vi "SetSamplingClockFrequency.vi"(1 "Sampling Clock Option":u16(ring) items=["Frequency Value", "Default", "Minimum", "Maximum"], 3 "error in (no error)":errorcluster, 4 "Sampling Clock (Hz)":dbl format="%#_16g", 5 "VISA resource name":refnum<visa-resource-name>) -> (0 "error out":errorcluster, 2 "VISA resource name out":refnum<visa-resource-name>)   [LabVIEW 2020, in "Active Technologies AWG3000.lvlib"]
uses:
  Active Technologies AWG3000.lvlib
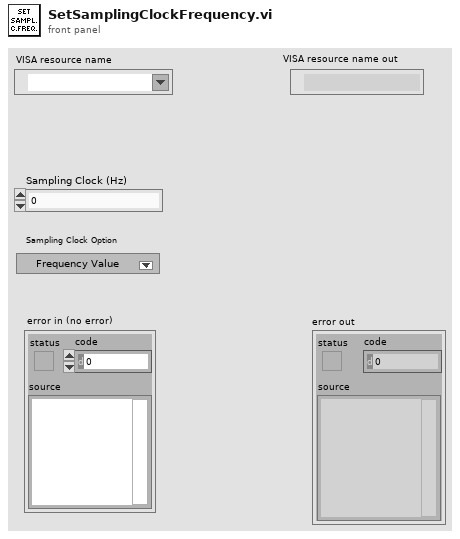
[diagram p1: front panel]
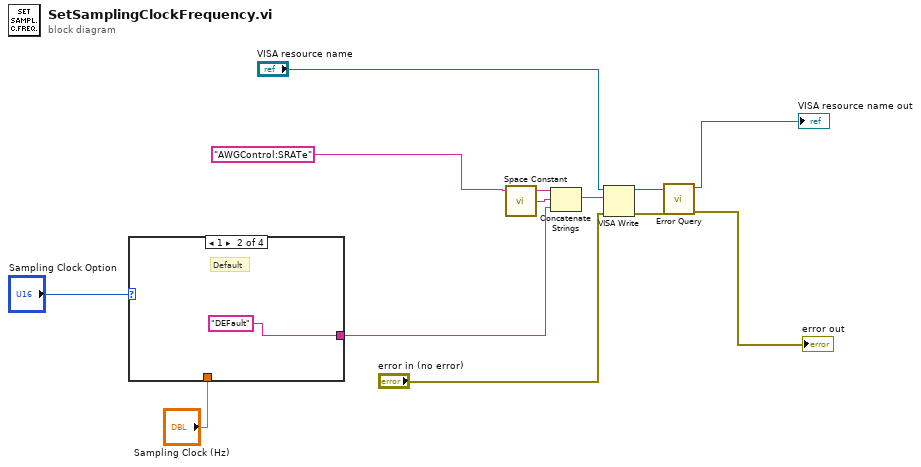
[diagram p0: block diagram]
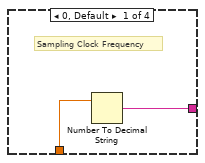
[diagram p2: hidden frame]
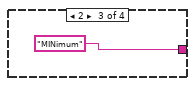
[diagram p3: hidden frame]
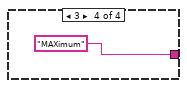
[diagram p4: hidden frame]
diagram:
  n1 = case shown="1" "Sampling Clock Option" {
    tunnel: [w14 "DEFault" ("write buffer") "MINimum" ("write buffer") "MAXimum" ("write buffer")] -> w3
    tunnel: "Sampling Clock (Hz)" -> [w13 _ _ _]
    frame 0, Default {
      # "Sampling Clock Frequency"
      n2 = Number To Decimal String(number=w13) -> (decimal integer string=w14:string)  [unwired: 1 in]
    }
    frame 1 {
      # "Default"
    }
    frame 2 {
    }
    frame 3 {
    }
  }
  n3 = call <vilib>:"Space Constant.vi"() -> ("String"=w6:string)
  n4 = Concatenate Strings("AWGControl:SRATe" ("write buffer"), w6, w3) -> (w5:string)
  n5 = VISA Write(VISA resource name="VISA resource name", write buffer=w5, error in (no error)="error in (no error)") -> (VISA resource name out=w10:refnum<visa-resource-name>, error out=w9:errorcluster)  [unwired: 1 out]
  n6 = call "Error Query.vi"("error in (no error)"=w9, "VISA resource name"=w10) -> ("error out"=→"error out":errorcluster, "VISA resource name out"=→"VISA resource name out":refnum<visa-resource-name>)  [unwired: 6 in, 2 out]
